vi "Pitch Offset To Decimal.vi"(11 "Pitch Offset (%)":dbl) -> (3 "Pitch (decimal)":dbl)   [LabVIEW 2019, in "Audio Processing.lvlib"]
doc: "Convert pitch offset (-30% to 30%) into decimal notation (0.7 to 1.3)."
uses:
  Audio Processing.lvlib
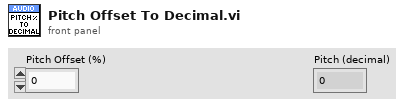
[diagram p1: front panel]
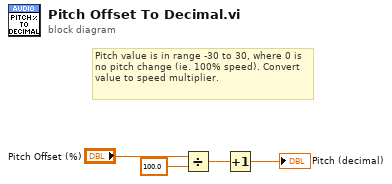
[diagram p0: block diagram]
diagram:
  # "Pitch value is in range -30 to 30, where 0 is no pitch change (ie. 100% speed). Convert value to speed multiplier."
  n1 = Divide(x="Pitch Offset (%)", y=100.0) -> (x/y=w3:dbl)
  n2 = Increment(x=w3) -> (x+1=→"Pitch (decimal)":dbl)
